vi "FMI_CH1.vi"(2 "Accel":i32=100, 3 "Direction":enum16{"Forward", "Reverse"}(ring), 4 "RPM":i32=375, 6 "Strokes":i32=3, 7 "Home Pump":bool) -> ()   [LabVIEW 2019]
uses:
  C:/Users/MUSE_V2/Desktop/CLIO/ConfigFiles/FMI_labview/FMI_LIB.dll
  ConfigFiles/FMI_labview/FMI_LIB.dll
panel:
  in  "ProgressBar?":bool
  out "Stroke#":dbl format="%#_4g"
  out "Step Completion (%)":dbl=100.91556705865854
  out "Pumping Progress":dbl(slide)=1.0091556705865854 scale=0.0..1.0
  in  "VISA resource name":refnum<visa-resource-name>="COM4"
  out "FMI_Connect":bool
  out "FMI_Disconnect":bool=TRUE
  out "Pump Runtime (s)":dbl=2.0094395102393197
  out "Pump Start":bool=TRUE
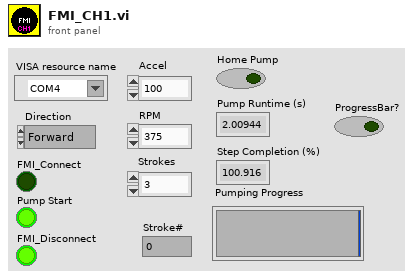
[diagram p1: front panel]
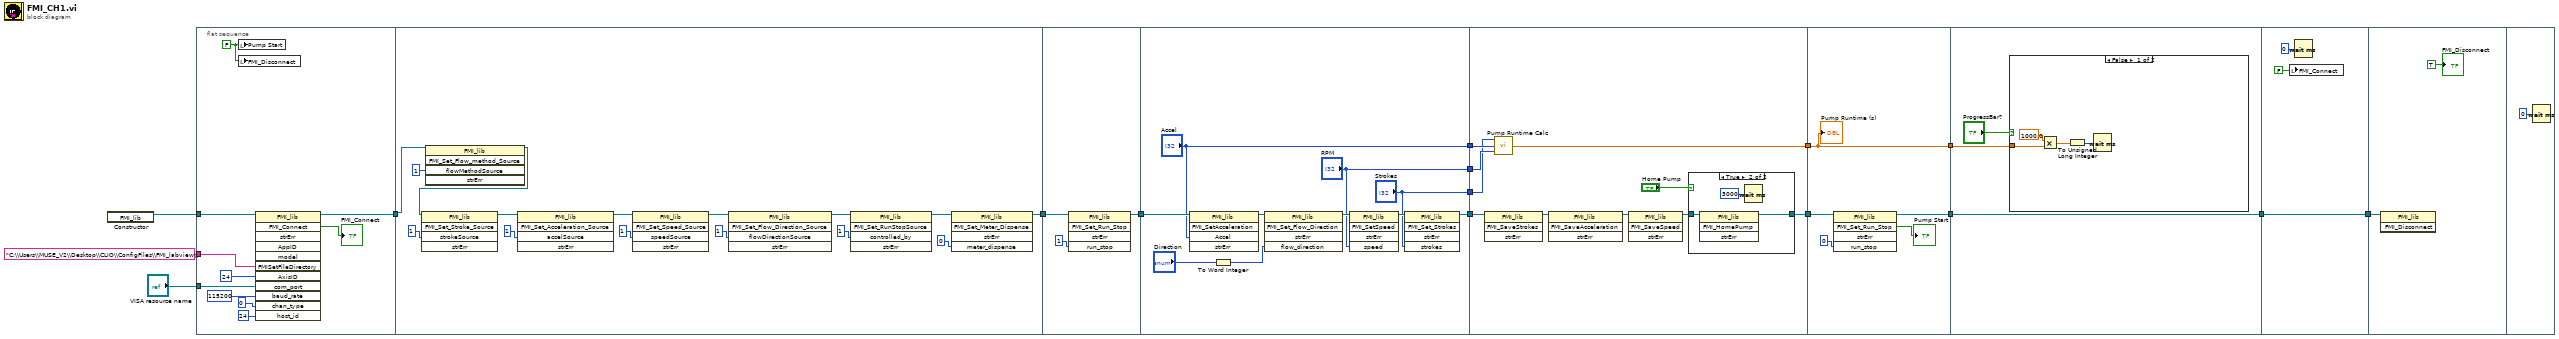
[diagram p0: block diagram]
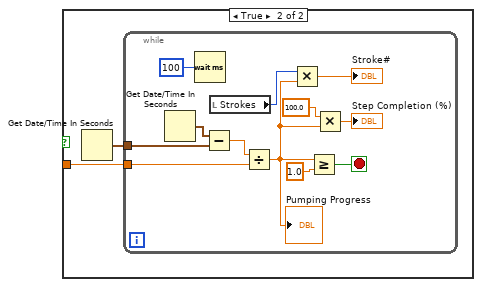
[diagram p3: hidden frame]
diagram:
  n1 = constructor class="FMI_lib"() -> (reference out=w16:refnum<k24>)  [unwired: 3 in, 2 out]
  n2 = flat-sequence {
    tunnel: [w23] -> w14
    tunnel: w16 -> [w26]
    tunnel: "C:\\Users\\MUSE_V2\\Desktop\\CLIO\\ConfigFiles\\FMI_labview\\" ("Path to setup files") -> [w24]
    tunnel: "VISA resource name" -> [w17]
    tunnel: w14 -> [w29]
    tunnel: [w30] -> w13
    tunnel: w13 -> [w43]
    tunnel: [w42] -> w12
    tunnel: w12 -> [w54]
    tunnel: [w50] -> w11
    tunnel: ["Accel"] -> w10
    tunnel: ["RPM"] -> w9
    tunnel: ["Strokes"] -> w8
    tunnel: w11 -> [w64]
    tunnel: [w56] -> w7
    tunnel: w10 -> [w61]
    tunnel: w9 -> [w60]
    tunnel: w8 -> [w59]
    tunnel: [w58] -> w6
    tunnel: w7 -> [w72]
    tunnel: [w71] -> w5
    tunnel: [w69] -> w4
    tunnel: w6 -> [w69]
    tunnel: [w76] -> w3
    tunnel: w5 -> [w76]
    tunnel: w4 -> [w75]
    tunnel: w3 -> [w97]
    tunnel: [w97] -> w2
    tunnel: w2 -> [w99]
    frame #0 {
      w21 = FALSE
      n3 = local write "Pump Start"(w21) -> ()
      n4 = local write "FMI_Disconnect"(w21) -> ()
      n5 = invoke class="FMI_lib" method="FMI_Connect"(reference=w26, "FMISetFileDirectory"=w24, "AxisID"=u8 24, "com_port"=w17, "baud_rate"=u32 115200, "chan_type"=u8 0, "host_id"=u8 24) -> (reference out=w23:refnum<k24>, "FMI_Connect"=→"FMI_Connect":bool)  [unwired: 5 in, 10 out]
    }
    frame #1 {
      n6 = invoke class="FMI_lib" method="FMI_Set_Flow_method_Source"(reference=w29, "flowMethodSource"=i16 1) -> (reference out=w28:refnum<k24>)  [unwired: 3 in, 4 out]
      n7 = invoke class="FMI_lib" method="FMI_Set_Stroke_Source"(reference=w28, "strokeSource"=i16 1) -> (reference out=w37:refnum<k24>)  [unwired: 3 in, 4 out]
      n8 = invoke class="FMI_lib" method="FMI_Set_Acceleration_Source"(reference=w37, "accelSource"=i16 1) -> (reference out=w36:refnum<k24>)  [unwired: 3 in, 4 out]
      n9 = invoke class="FMI_lib" method="FMI_Set_Speed_Source"(reference=w36, "speedSource"=i16 1 ("strokeSource")) -> (reference out=w35:refnum<k24>)  [unwired: 3 in, 4 out]
      n10 = invoke class="FMI_lib" method="FMI_Set_Flow_Direction_Source"(reference=w35, "flowDirectionSource"=i16 1) -> (reference out=w34:refnum<k24>)  [unwired: 3 in, 4 out]
      n11 = invoke class="FMI_lib" method="FMI_Set_RunStopSource"(reference=w34, "controlled_by"=i16 1) -> (reference out=w31:refnum<k24>)  [unwired: 3 in, 4 out]
      n12 = invoke class="FMI_lib" method="FMI_Set_Meter_Dispense"(reference=w31, "meter_dispense"=i16 0) -> (reference out=w30:refnum<k24>)  [unwired: 3 in, 4 out]
    }
    frame #2 {
      n13 = invoke class="FMI_lib" method="FMI_Set_Run_Stop"(reference=w43, "run_stop"=i16 1) -> (reference out=w42:refnum<k24>)  [unwired: 3 in, 4 out]
    }
    frame #3 {
      n14 = invoke class="FMI_lib" method="FMI_SetAcceleration"(reference=w54, "Accel"="Accel") -> (reference out=w53:refnum<k24>)  [unwired: 3 in, 4 out]
      n15 = To Word Integer(number="Direction") -> (16bit integer=w45:i16)
      n16 = invoke class="FMI_lib" method="FMI_Set_Flow_Direction"(reference=w53, "flow_direction"=w45) -> (reference out=w52:refnum<k24>)  [unwired: 3 in, 4 out]
      n17 = invoke class="FMI_lib" method="FMI_SetSpeed"(reference=w52, "speed"="RPM") -> (reference out=w51:refnum<k24>)  [unwired: 3 in, 4 out]
      n18 = invoke class="FMI_lib" method="FMI_Set_Strokes"(reference=w51, "strokes"="Strokes") -> (reference out=w50:refnum<k24>)  [unwired: 3 in, 4 out]
    }
    frame #4 {
      n19 = invoke class="FMI_lib" method="FMI_SaveStrokes"(reference=w64) -> (reference out=w63:refnum<k24>)  [unwired: 3 in, 3 out]
      n20 = call "Pump Runtime Calc.vi"("RPM"=w60, "Accel"=w61, "Strokes"=w59) -> ("Pump Runtime (s)"=w58:dbl)
      n21 = invoke class="FMI_lib" method="FMI_SaveAcceleration"(reference=w63) -> (reference out=w62:refnum<k24>)  [unwired: 3 in, 3 out]
      n22 = invoke class="FMI_lib" method="FMI_SaveSpeed"(reference=w62) -> (reference out=w57:refnum<k24>)  [unwired: 3 in, 3 out]
      n23 = case shown="True" "Home Pump" {
        tunnel: w57 -> [w65 w68]
        tunnel: [w65 w67] -> w56
        frame False {
        }
        frame True {
          n24 = invoke class="FMI_lib" method="FMI_HomePump"(reference=w68) -> (reference out=w67:refnum<k24>)  [unwired: 3 in, 3 out]
          n25 = Wait (ms)(milliseconds to wait=u32 3000) -> ()  [unwired: 1 out]
        }
      }
    }
    frame #5 {
      n26 = invoke class="FMI_lib" method="FMI_Set_Run_Stop"(reference=w72, "run_stop"=i16 0) -> (reference out=w71:refnum<k24>, "FMI_Set_Run_Stop"=→"Pump Start":bool)  [unwired: 3 in, 3 out]
      "Pump Runtime (s)" <- w69
    }
    frame #6 {
      n27 = case shown="False" "ProgressBar?" {
        tunnel: w75 -> [w80 w81]
        frame False {
          n28 = Multiply(x=1000.0, y=w80) -> (x*y=w78:dbl)
          n29 = To Unsigned Long Integer(number=w78) -> (unsigned 32bit integer=w77:u32)
          n30 = Wait (ms)(milliseconds to wait=w77) -> ()  [unwired: 1 out]
        }
        frame True {
          n31 = Get Date/Time In Seconds() -> (seconds since 1Jan1904=w82:timestamp)
          n32 = while {
            tunnel: w82 -> [w92]
            tunnel: w81 -> [w89]
            stop <- w93 stop-if-true
            n33 = Get Date/Time In Seconds() -> (seconds since 1Jan1904=w90:timestamp)
            n34 = Wait (ms)(milliseconds to wait=u32 100) -> ()  [unwired: 1 out]
            n35 = Subtract(x=w90, y=w92) -> (x-y=w91:dbl)
            n36 = local read "Strokes"() -> (w84:i32)
            n37 = Divide(x=w91, y=w89) -> (x/y=w85:dbl)
            "Pumping Progress" <- w85
            n38 = Multiply(x=w84, y=w85) -> (x*y=→"Stroke#":dbl)
            n39 = Greater Or Equal?(x=w85, y=1.0) -> (x >= y?=w93:bool)
            n40 = Multiply(x=100.0, y=w85) -> (x*y=→"Step Completion (%)":dbl)
          }
        }
      }
    }
    frame #7 {
      n41 = local write "FMI_Connect"(FALSE) -> ()
      n42 = Wait (ms)(milliseconds to wait=u32 0) -> ()  [unwired: 1 out]
    }
    frame #8 {
      n43 = invoke class="FMI_lib" method="FMI_Disconnect"(reference=w99) -> ()  [unwired: 2 in, 3 out]
      "FMI_Disconnect" <- TRUE
    }
    frame #9 {
      n44 = Wait (ms)(milliseconds to wait=u32 0) -> ()  [unwired: 1 out]
    }
  }
